vi "Asylum_SendIgorCommand.vi"(8 "error in (no error)":errorcluster, 9 "Format":string, 10 "command":string, 11 "Application In":refnum<k7>) -> (0 "error out":errorcluster, 1 "history":string, 2 "results":string, 3 "Application Out":refnum<k7>)   [LabVIEW 2020]
uses:
  3e75c103-e1b9-4305-8c72-ede530a43926.vi
  3e75c103-e1b9-4305-8c72-ede530a43926.vi/ff40df25-0e41-4205-825d-56c19dc320b6.vi
  <vilib>/Utility/Debug Log/Display.vi
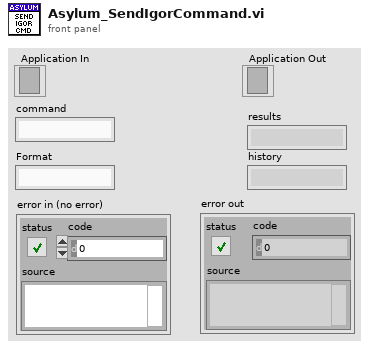
[diagram p1: front panel]
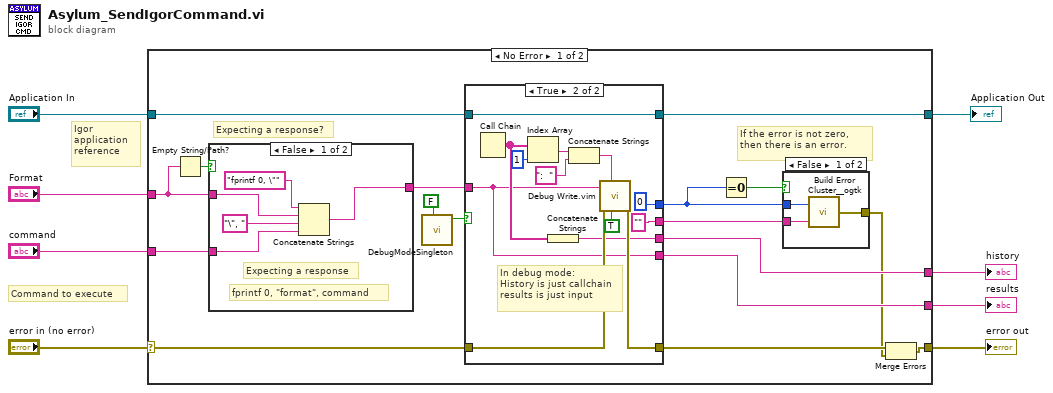
[diagram p0: block diagram]
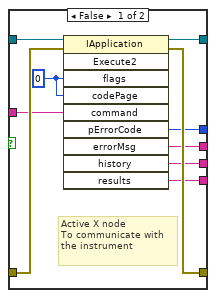
[diagram p2: hidden frame]
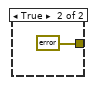
[diagram p4: hidden frame]
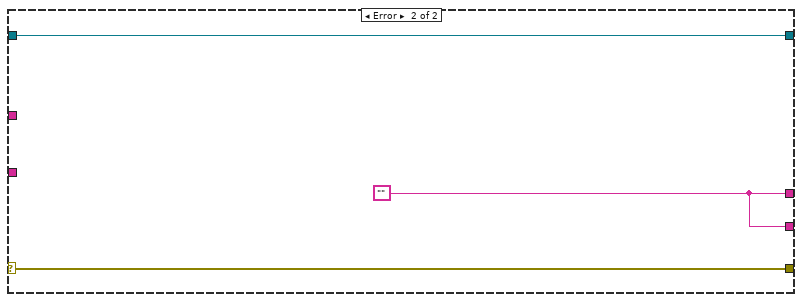
[diagram p5: hidden frame]
diagram:
  # "Command to execute"
  # "Igor application reference"
  n1 = case shown="No Error" "error in (no error)" {
    selector: "error in (no error)" -> [w25 w61]
    tunnel: [w23 w61] -> w8
    tunnel: "Application In" -> [w22 w60]
    tunnel: "command" -> [w13 _]
    tunnel: [w18 w59] -> w4
    tunnel: [w17 w59] -> w3
    tunnel: [w16 w60] -> w2
    tunnel: "Format" -> [w12 _]
    frame No Error {
      # "Expecting a response?"
      # "If the error is not zero, then there is an error."
      n2 = Empty String/Path?(string/path=w12) -> (empty?=w15:bool)
      n3 = case shown="False" w15 {
        tunnel: [w49 w54] -> w14
        tunnel: w13 -> [w50 w54]
        tunnel: w12 -> [w52 _]
        frame False {
          # "Expecting a response"
          # "fprintf 0, \"format\", command"
          n4 = Concatenate Strings("fprintf 0, \"" ("string"), w52, "\", " ("string"), w50) -> (w49:string)
        }
        frame True {
          # "Not expecting a response"
          # "Command"
        }
      }
      n5 = call "DebugModeSingleton.vi"("Write?"=FALSE) -> ("Debug Mode?"=w11:bool)  [unwired: 10 in]
      n6 = case shown="True" w11 {
        tunnel: w22 -> [w33 w44]
        tunnel: w25 -> [w35 w48]
        tunnel: [w31 0] -> w20
        tunnel: [w30 "" ("errorMsg")] -> w19
        tunnel: [w34 w47] -> w24
        tunnel: [w29 w37] -> w18
        tunnel: [w28 w36] -> w17
        tunnel: [w27 w44] -> w16
        tunnel: w14 -> [w26 w36]
        frame False {
          w32 = 0 ("flags")
          # "Active X node\nTo communicate with the instrument"
          n7 = invoke on="Invoke Node" class="IApplication" method="Execute2"(reference=w33, error in=w35, "flags"=w32, "codePage"=w32, "command"=w26) -> (reference out=w27:refnum<k7>, error out=w34:errorcluster, "pErrorCode"=w31:i32, "errorMsg"=w30:string, "history"=w29:string, "results"=w28:string)  [unwired: 5 in, 4 out]
        }
        frame True {
          # "In debug mode:\nHistory is just callchain\nresults is just input"
          n8 = Call Chain() -> (call chain=w38:string[])
          n9 = Index Array(array=w38, index=1) -> (element=w42:string)
          n10 = Concatenate Strings(w38) -> (w37:string)
          n11 = Concatenate Strings(w42, ":  " ("string")) -> (w41:string)
          n12 = call "Debug Write.vim"("include timestamp? (F)"=TRUE, "prefix (\"\")"=w41, "error in (no error)"=w48, "value"=w36) -> ("error out"=w47:errorcluster)  [unwired: 7 in]
        }
      }
      n13 = Equal To 0?(x=w20) -> (x = 0?=w21:bool)
      n14 = case shown="False" w21 {
        tunnel: w20 -> [w56 _]
        tunnel: w19 -> [w55 _]
        tunnel: [w57 errorcluster {"status"=FALSE, "code"=0, "source"=""} ("error constant")] -> w9
        frame False {
          n15 = call <userlib>:"Build Error Cluster__ogtk.vi"("String to Prepend to source (\"\")"=w55, "code"=w56) -> ("error out"=w57:errorcluster)
        }
        frame True {
        }
      }
      n16 = Merge Errors(w24, w9) -> (w23:errorcluster)
    }
    frame Error {
      w59 = ""
    }
  }
  "error out" <- w8
  "history" <- w4
  "results" <- w3
  "Application Out" <- w2
